vi "CLD 9 Step Sequencer Express Timer Solution.vi"() -> ()   [LabVIEW 2009]
doc: "CLD 9\n\nDieses Lösungs-VI verwendet das Express-VI \"Verstrichene Zeit\" zum Messen der Zeit bei der Änderung von Zuständen. Alle statistischen Daten dieser Übung sind hardcodiert."
uses:
  CLD 9 Timer Enum.ctl
panel:
  out "Dauer des aktuellen Schritts":dbl
  out "Verstrichene Zeit (s)":dbl format="%#.1g"
  out "Schritt 3":bool
  out "Schritt 2":bool
  out "Schritt 1":bool
  out "Zeit ist verstrichen":bool
  in  "Autom. zurücksetzen":bool
  in  "Zurücksetzen-Schaltfläche":bool
  in  "VI anhalten":bool
  out "Fehler (Ausgang)":errorcluster
  in  "Fehler (Eingang)":errorcluster
  in  "Zielzeit (s)":dbl
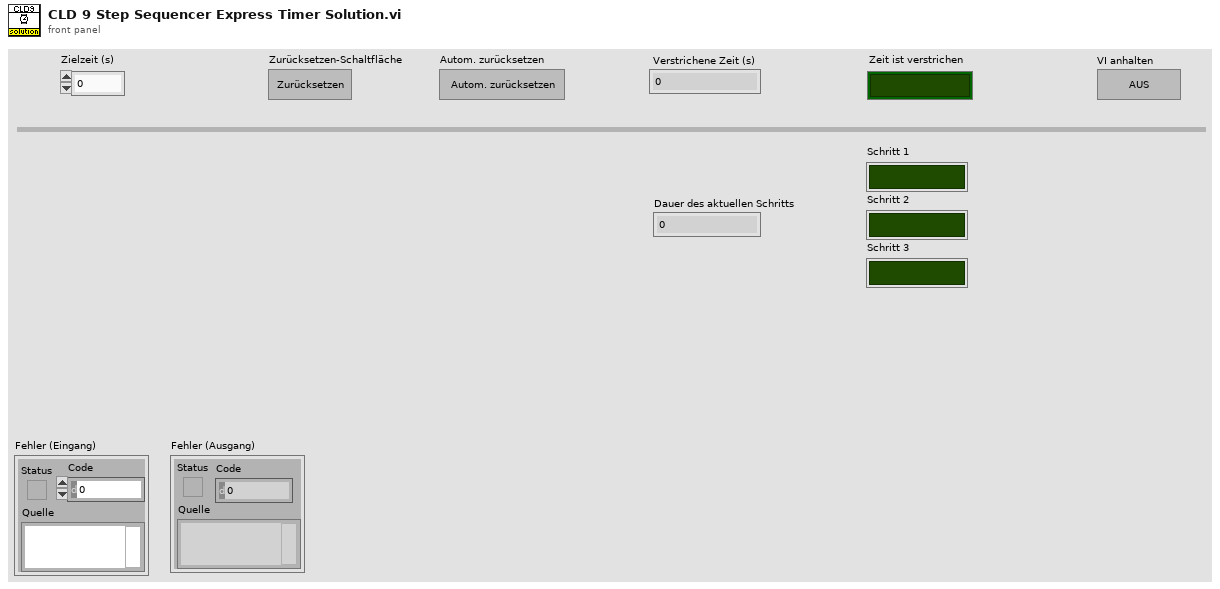
[diagram p1: front panel]
types:
  T1 = typedef "CLD 9 Timer Enum.ctl" = enum16{"Schritt eins ausführen", "Schritt zwei ausführen", "Schritt drei ausführen"}
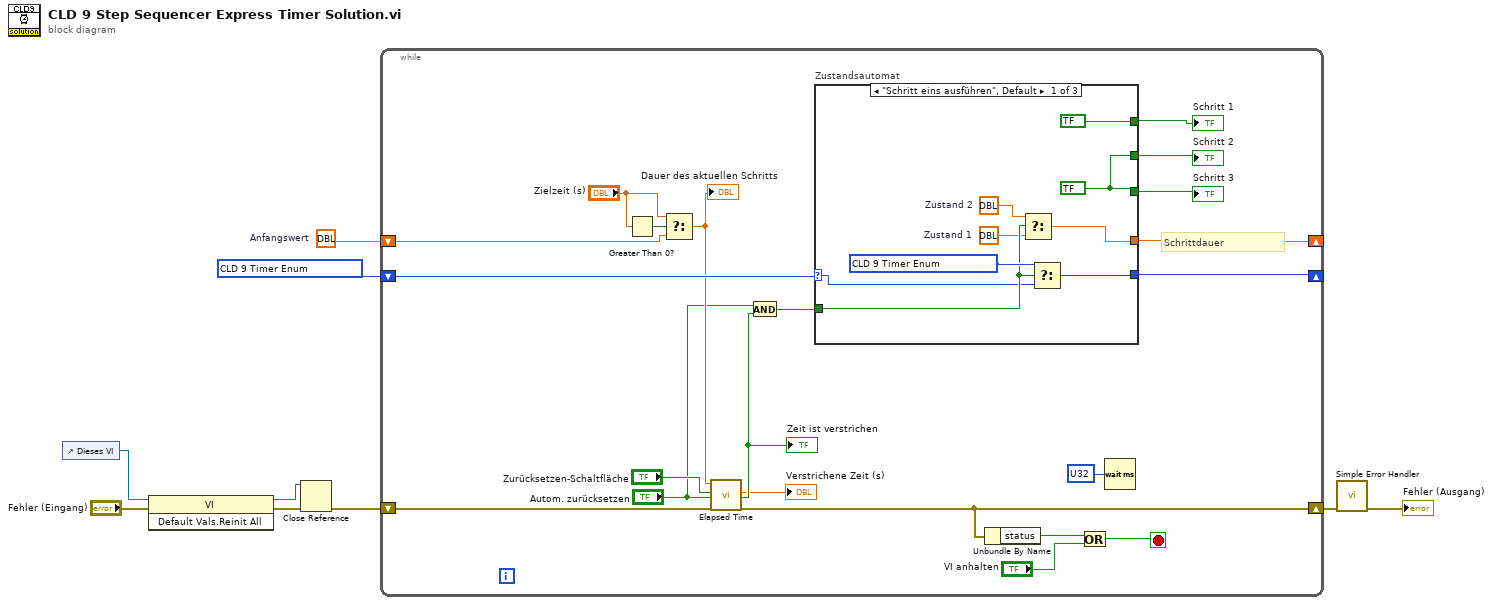
[diagram p0: block diagram]
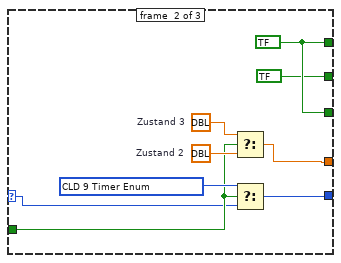
[diagram p2: hidden frame]
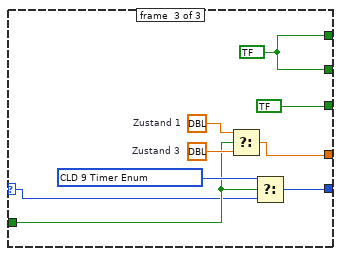
[diagram p3: hidden frame]
diagram:
  w1 = dbl ?  # Anfangswert
  n1 = control-ref of="Dieses VI"() -> (w5:refnum<vi>)
  n2 = invoke on="Invoke Node" class="VI" method="Default Vals.Reinit All"(reference=w5, error in="Fehler (Eingang)") -> (reference out=w3:refnum<vi>, error out=w6:errorcluster)  [unwired: 1 in, 1 out]
  n3 = Close Reference(reference=w3, error in (no error)=w6) -> (error out=w4:errorcluster)
  n4 = while {
    shift-right: [w13] -> w8
    shift-left: w4 -> [w28]
    shift-right: [w26] -> _
    shift-left: T1 ? ("Enum") -> [w25]
    shift-right: [w17] -> _
    shift-left: w1 -> [w16]
    stop <- w12 stop-if-true
    # "Schrittdauer"
    n5 = Greater Than 0?(x="Zielzeit (s)") -> (x > 0?=w20:bool)
    n6 = Select(t="Zielzeit (s)", s=w20, f=w16) -> (s? t:f=w18:dbl)
    "Dauer des aktuellen Schritts" <- w18
    n7 = call "Elapsed Time"("Time Target (s)"=w18, "Reset"="Zurücksetzen-Schaltfläche", "Auto Reset"="Autom. zurücksetzen", "error in (no error)"=w28) -> ("Elapsed Time (s)"=→"Verstrichene Zeit (s)":dbl, "Time has Elapsed"=w24:bool, "error out"=w13:errorcluster)  [unwired: 8 in, 5 out]
    "Zeit ist verstrichen" <- w24
    n8 = And(x="Autom. zurücksetzen", y=w24) -> (x .and. y?=w15:bool)
    n9 = case "Zustandsautomat" shown="\"Schritt eins ausführen\", Default" w25 {
      selector: w25 -> [w31 w40 w49]
      tunnel: [w36 w47 w56] -> w26
      tunnel: w15 -> [w35 w41 w50]
      tunnel: [bool ? w46 w54] -> w23
      tunnel: [w38 bool ? w54] -> w22
      tunnel: [w38 w46 bool ?] -> w21
      tunnel: [w32 w42 w51] -> w17
      frame #0 {
        w33 = dbl ?  # Zustand 1
        w34 = dbl ?  # Zustand 2
        w38 = bool ?
        n10 = Select(t=w34, s=w35, f=w33) -> (s? t:f=w32:dbl)
        n11 = Select(t=T1 ?, s=w35, f=w31) -> (s? t:f=w36:T1)
      }
      frame #1 {
        w43 = dbl ?  # Zustand 2
        w44 = dbl ?  # Zustand 3
        w46 = bool ?
        n12 = Select(t=w44, s=w41, f=w43) -> (s? t:f=w42:dbl)
        n13 = Select(t=T1 ?, s=w41, f=w40) -> (s? t:f=w47:T1)
      }
      frame #2 {
        w52 = dbl ?  # Zustand 3
        w53 = dbl ?  # Zustand 1
        w54 = bool ?
        n14 = Select(t=w53, s=w50, f=w52) -> (s? t:f=w51:dbl)
        n15 = Select(t=T1 ?, s=w50, f=w49) -> (s? t:f=w56:T1)
      }
    }
    "Schritt 1" <- w23
    "Schritt 2" <- w22
    "Schritt 3" <- w21
    n16 = Unbundle By Name(w13) -> ("status"=w11:bool)
    n17 = Or(x=w11, y="VI anhalten") -> (x .or. y?=w12:bool)
    n18 = Wait (ms)(milliseconds to wait=u32 ? ("Zu wartende ms")) -> ()  [unwired: 1 out]
  }
  n19 = call <vilib>:"Simple Error Handler.vi"("error in (no error)"=w8) -> ("error out"=→"Fehler (Ausgang)":errorcluster)  [unwired: 4 in, 4 out]
